vi "wavelength scan_v1.0.vi"() -> ()   [LabVIEW 2012]
panel:
  out "Power Chart":dbl(graph)=1.568e-05
  in  "range (0=auto)":i32
  in  "wavelength":i32=4
  in  "filter (0=out)":i32
  out "OfflineTEC_offset":dbl=-6.6023368 format="%#.4g"
  out "OnLineTEC_offset":dbl=-0.02357750000000003 format="%.4g"
  in  "offlineTEC_offset":dbl format="%.4g"
  in  "onlineTEC_offset":dbl format="%.4g"
  out "Lambda Read (nm)":dbl=780.2608522506264 format="%.5f"
  out "Wavelength Lock":bool=TRUE
  out "XY Graph":cluster{"Y":dbl[], "Y":dbl[]}[](graph)
  in  "Online":bool=TRUE
  out "Power (W)":dbl=1.568e-05 format="%.3p"
  out "OphirPM":T1={"Ophir-Ref"=refnum, "Ophir-Device"=1000, "Ophir-Channel"=0}
  out "Waveform Chart":dbl(graph)=780.2608522506264
  in  "Lambda Step (nm)":dbl=5e-05 format="%.5f"
  in  "Lambda Stop (nm)":dbl=780.261 format="%.5f"
  in  "Lambda Start (nm)":dbl=780.231 format="%.5f"
  in  "step_size":dbl=0.001 format="%#_6p"
  in  "Device In":refnum<visa-resource-name>="Pro8000"
  in  "Settings":T2={"Module"=enum."On Line TEC", "OnLineTEC"=14.05, "OnLineLD"=0.16, "OffLineTEC"=29.538, "OffLineLD"=0.173, "EtalonTEC"=27.0, "TSOA-TEC"=19.0} {"OffLineLD" min=0.0 max=0.175 step=0.001 format="%.3p"; "OnLineLD" min=0.0 max=0.175 step=0.001 format="%.3p"; "TSOA-TEC" format="%.2g"; "EtalonTEC" format="%.2g"; "OffLineTEC" min=0.0 max=30.0 step=0.1 format="%.3g"; "OnLineTEC" min=0.0 max=30.0 step=0.1 format="%.3g"}
  out "Readings":T3={"OnLineTEC"=14.0264225, "OnLineLD"=0.160541028, "OffLineTEC"=22.9356632, "OffLineLD"=0.000128906249, "EtalonTEC"=28.0260735, "TSOA-TEC"=19.0028629, "Pro8000"=TRUE, "OnLine TEC"=TRUE, "OnLine LD"=TRUE, "OffLine TEC"=FALSE, "OffLine LD"=FALSE, "Etalon TEC"=TRUE, "TSOA TEC"=TRUE} {"OffLineLD" format="%.4g"; "OnLineLD" format="%.4g"; "TSOA-TEC" format="%.3g"; "EtalonTEC" format="%.3g"; "OffLineTEC" format="%.3g"; "OnLineTEC" format="%.3g"}
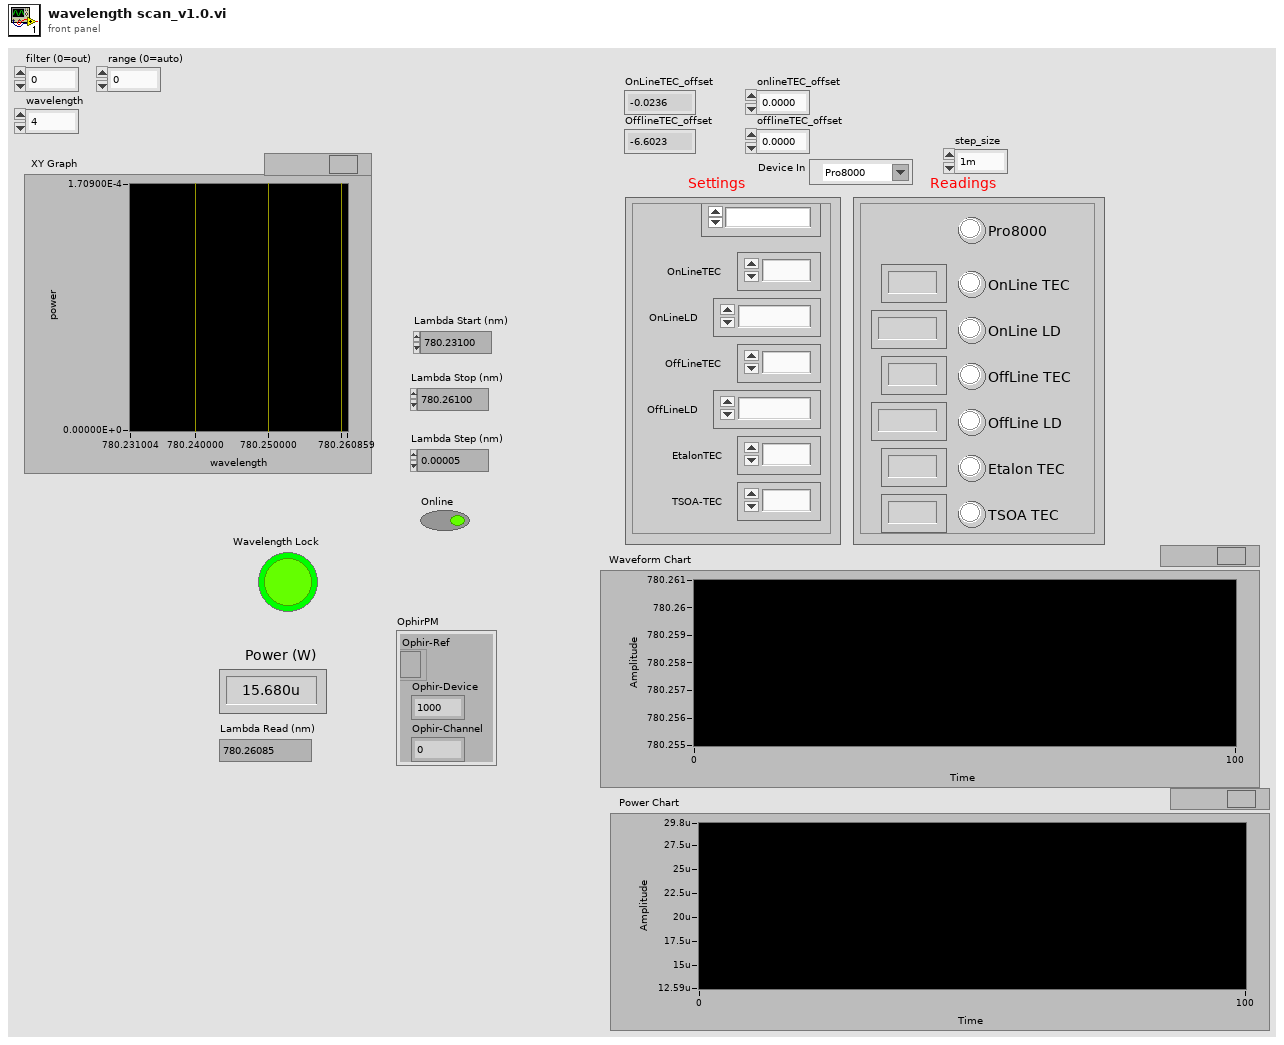
[diagram p1: front panel]
types:
  T1 = cluster{"Ophir-Ref":refnum<k7>, "Ophir-Device":i32, "Ophir-Channel":i32}
  T2 = cluster{"Module":enum16{"On Line TEC", "On Line LD", "Off Line TEC", "Off Line LD", "Etalon TEC", "TSOA TEC"}, "OnLineTEC":dbl, "OnLineLD":dbl, "OffLineTEC":dbl, "OffLineLD":dbl, "EtalonTEC":dbl, "TSOA-TEC":dbl}
  T3 = cluster{"OnLineTEC":dbl, "OnLineLD":dbl, "OffLineTEC":dbl, "OffLineLD":dbl, "EtalonTEC":dbl, "TSOA-TEC":dbl, "Pro8000":bool, "OnLine TEC":bool, "OnLine LD":bool, "OffLine TEC":bool, "OffLine LD":bool, "Etalon TEC":bool, "TSOA TEC":bool}
  T4 = enum16{"On Line TEC", "On Line LD", "Off Line TEC", "Off Line LD", "Etalon TEC", "TSOA TEC"}
  T5 = enum16{"Open_TL", "Close_TL", "Verify_ID", "TEC_Sensor", "SET", "READ", "ON", "OFF", "Set_Limits", "Read_Limits", "Enable_Status", "Read_Status"}
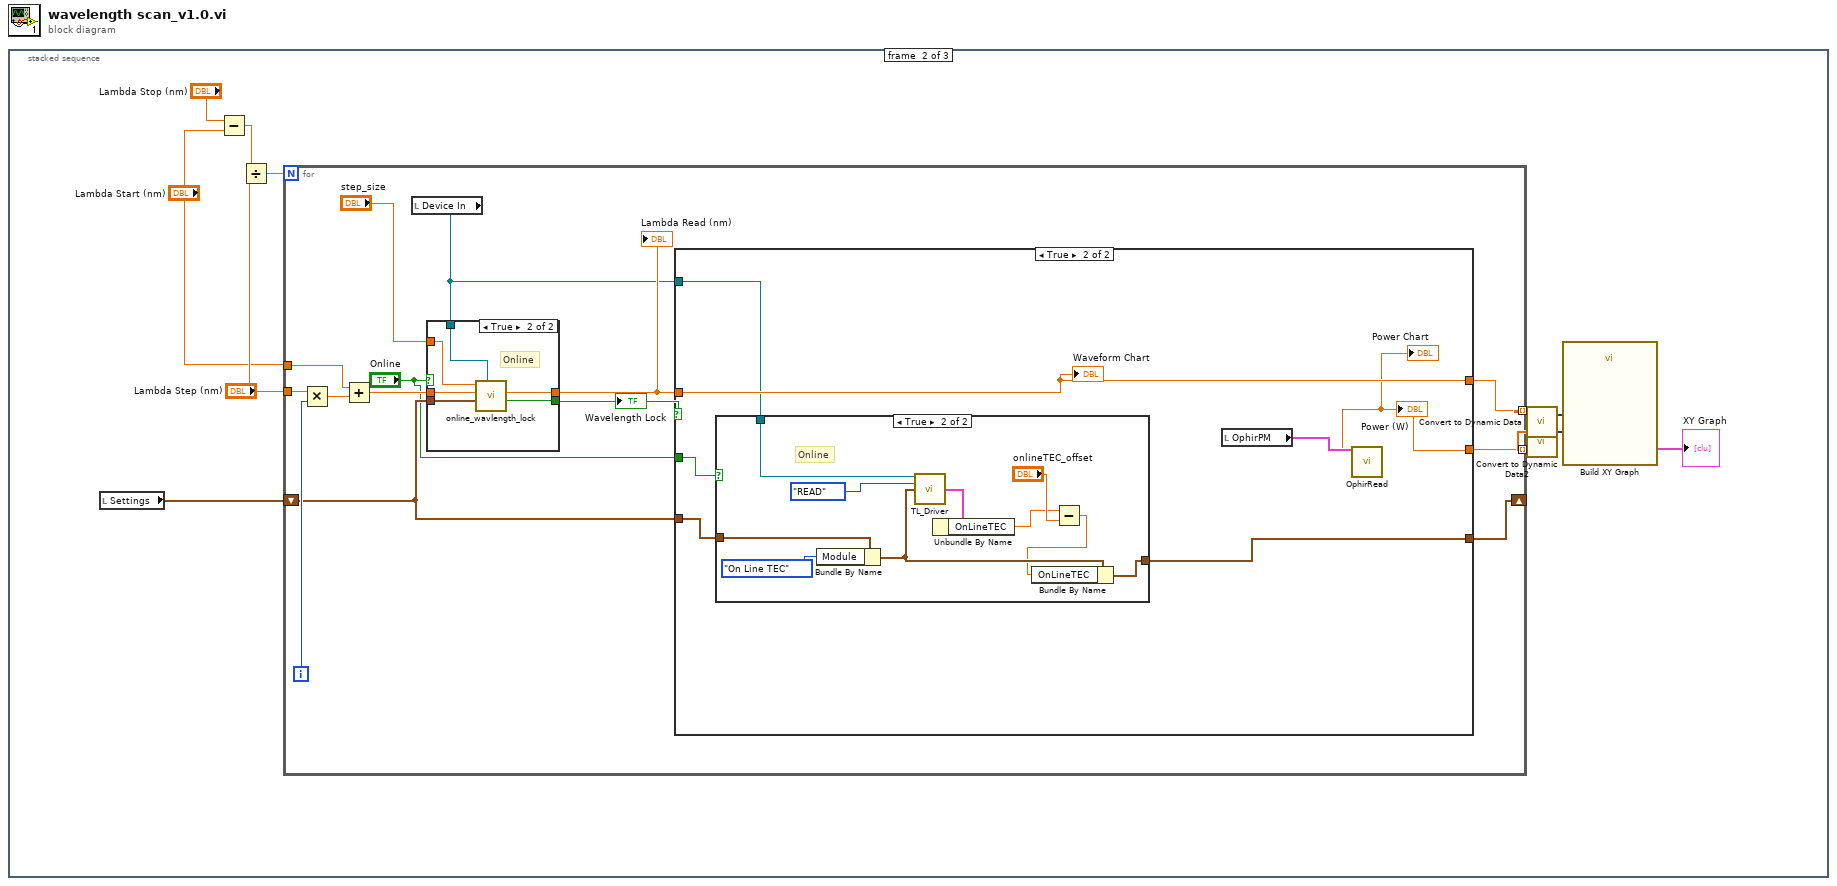
[diagram p0: block diagram]
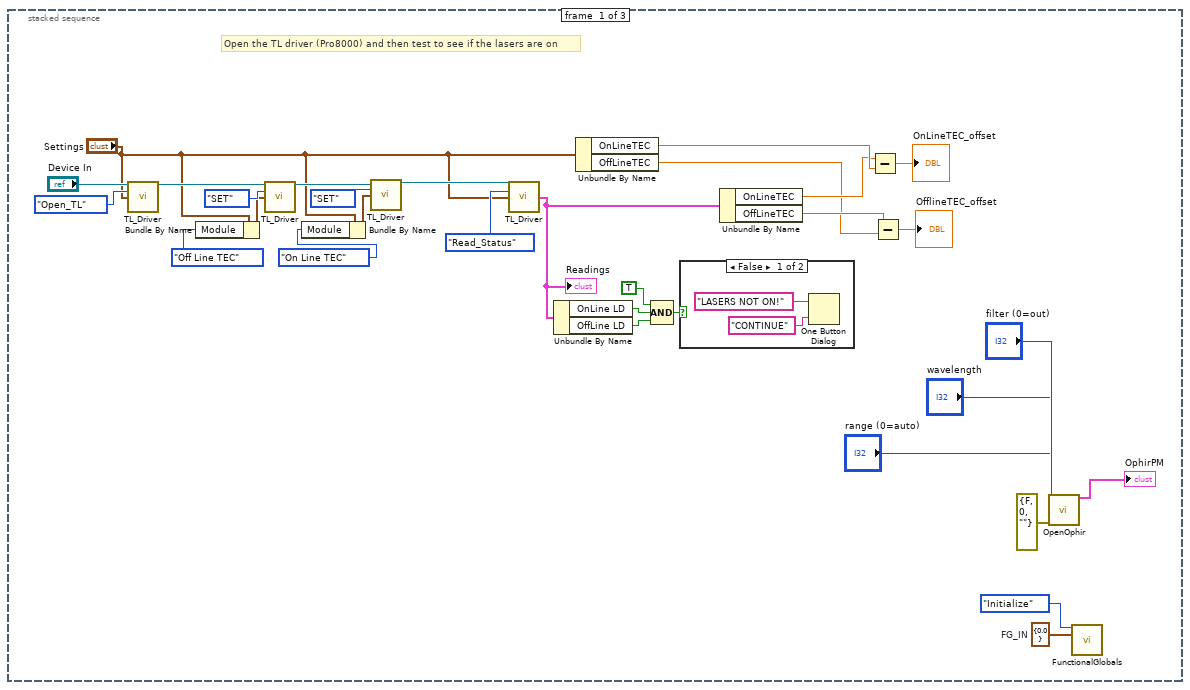
[diagram p2: hidden frame]
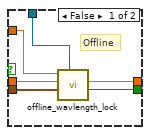
[diagram p4: hidden frame]
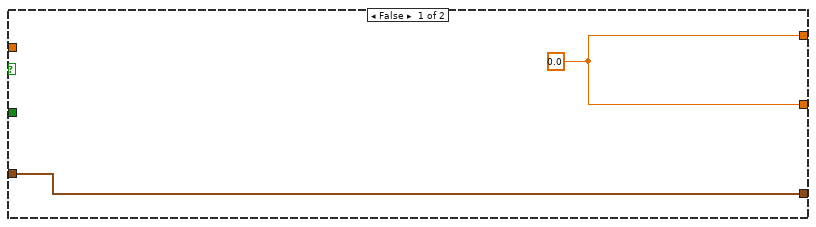
[diagram p5: hidden frame]
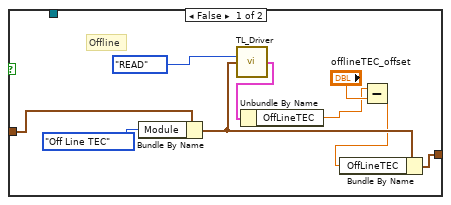
[diagram p6: hidden frame]
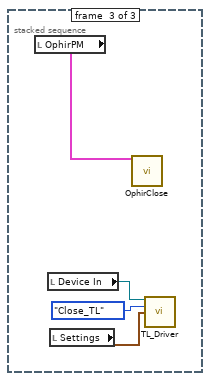
[diagram p7: hidden frame]
diagram:
  n1 = stacked-sequence {
    frame #0 {
      w22 = cluster{"PowerIn":dbl} {"PowerIn"=0.0}  # FG_IN
      # "Open the TL driver (Pro8000) and then test to see if the lasers are on"
      n2 = call "TL_Driver.vi"("Device In"="Device In", "Commands"=T5."Open_TL", "Settings"="Settings") -> ("Device Out"=w18:refnum<visa-resource-name>)  [unwired: 9 in, 3 out]
      n3 = Bundle By Name(cluster="Settings", "Module"=T4."Off Line TEC") -> (w15:T2)
      n4 = call "TL_Driver.vi"("Device In"=w18, "Commands"=T5."SET", "Settings"=w15) -> ("Device Out"=w13:refnum<visa-resource-name>)  [unwired: 9 in, 3 out]
      n5 = Bundle By Name(cluster="Settings", "Module"=T4."On Line TEC") -> (w14:T2)
      n6 = call "TL_Driver.vi"("Device In"=w13, "Commands"=T5."SET", "Settings"=w14) -> ("Device Out"=w12:refnum<visa-resource-name>)  [unwired: 9 in, 3 out]
      n7 = call "TL_Driver.vi"("Device In"=w12, "Commands"=T5."Read_Status", "Settings"="Settings") -> ("Readings"=w4:T3)  [unwired: 9 in, 3 out]
      "Readings" <- w4
      n8 = Unbundle By Name(w4) -> ("OnLine LD"=w29:bool, "OffLine LD"=w28:bool)
      n9 = Unbundle By Name("Settings") -> ("OnLineTEC"=w8:dbl, "OffLineTEC"=w5:dbl)
      n10 = Compound Arithmetic op=AND(TRUE, w29, w28) -> (w30:bool)
      n11 = case shown="False" w30 {
        frame False {
          n12 = One Button Dialog(message="LASERS NOT ON!", button name ("OK")="CONTINUE") -> ()  [unwired: 1 out]
        }
        frame True {
        }
      }
      n13 = Unbundle By Name(w4) -> ("OnLineTEC"=w7:dbl, "OffLineTEC"=w6:dbl)
      n14 = Subtract(x=w7, y=w8) -> (x-y=→"OnLineTEC_offset":dbl)
      n15 = Subtract(x=w6, y=w5) -> (x-y=→"OfflineTEC_offset":dbl)
      n16 = call "OpenOphir.vi"("filter (0=out)"="filter (0=out)", "wavelength"="wavelength", "range (0=auto)"="range (0=auto)", "error in (no error)"=errorcluster {"status"=FALSE, "code"=0, "source"=""}) -> ("OphirPM"=→"OphirPM":T1)  [unwired: 10 in, 1 out]
      n17 = call "FunctionalGlobals.vi"("FG_Control"=enum16{"Initialize", "PowerRead", "PowerWrite"}."Initialize", "FG_IN"=w22) -> ()  [unwired: 13 in, 1 out]
    }
    frame #1 {
      n18 = local read "Settings"() -> (w34:T2)
      n19 = Subtract(x="Lambda Stop (nm)", y="Lambda Start (nm)") -> (x-y=w44:dbl)
      n20 = Divide(x=w44, y="Lambda Step (nm)") -> (x/y=w43:dbl)
      n21 = for {
        N: w43 -> [_]
        tunnel: "Lambda Step (nm)" -> [w57]
        tunnel: "Lambda Start (nm)" -> [w56]
        tunnel: [w52] -> w38 mode=indexing
        tunnel: [w51] -> w36 mode=indexing
        shift-right: [w48] -> _
        shift-left: w34 -> [w46]
        i -> [w58]
        n22 = Multiply(x=w57, y=w58) -> (x*y=w55:dbl)
        n23 = Add(x=w56, y=w55) -> (x+y=w54:dbl)
        n24 = local read "Device In"() -> (w47:refnum<visa-resource-name>)
        n25 = case shown="True" "Online" {
          tunnel: w54 -> [w62 w70]
          tunnel: w47 -> [w63 w69]
          tunnel: w46 -> [w61 w68]
          tunnel: [w60 w67] -> w50
          tunnel: [w59 w66] -> w49
          tunnel: "step_size" -> [w64 w65]
          frame False {
            # "Offline"
            n26 = call "offline_wavlength_lock.vi"("Device"=w63, "Settings In"=w61, "Lambda Off Set (nm)"=w62, "step_size"=w64) -> ("Wavelength Lock Offline"=w60:bool, "Lambda Off Read (nm)"=w59:dbl)  [unwired: 3 in]
          }
          frame True {
            # "Online"
            n27 = call "online_wavlength_lock.vi"("Device"=w69, "Settings In"=w68, "Lambda On Set (nm)"=w70, "step_size"=w65) -> ("Wavelength Lock Online"=w67:bool, "Lambda On Read (nm)"=w66:dbl)  [unwired: 3 in]
          }
        }
        "Wavelength Lock" <- w50
        "Lambda Read (nm)" <- w49
        n28 = case shown="True" w50 {
          tunnel: w49 -> [_ w78]
          tunnel: [w72 w78] -> w52
          tunnel: [w72 w73] -> w51
          tunnel: [w71 w74] -> w48
          tunnel: w47 -> [_ w77]
          tunnel: w46 -> [w71 w76]
          tunnel: "Online" -> [_ w75]
          frame False {
            w72 = 0.0
          }
          frame True {
            n29 = case shown="True" w75 {
              tunnel: w77 -> [_ w97]
              tunnel: w76 -> [w87 w96]
              tunnel: [w83 w92] -> w74
              frame False {
                # "Offline"
                n30 = Bundle By Name(cluster=w87, "Module"=T4."Off Line TEC") -> (w84:T2)
                n31 = call "TL_Driver.vi"("Commands"=T5."READ", "Settings"=w84) -> ("Readings"=w85:T3)  [unwired: 10 in, 3 out]
                n32 = Unbundle By Name(w85) -> ("OffLineTEC"=w81:dbl)
                n33 = Subtract(x=w81, y="offlineTEC_offset") -> (x-y=w80:dbl)
                n34 = Bundle By Name(cluster=w84, "OffLineTEC"=w80) -> (w83:T2)
              }
              frame True {
                # "Online"
                n35 = Bundle By Name(cluster=w96, "Module"=T4."On Line TEC") -> (w93:T2)
                n36 = call "TL_Driver.vi"("Device In"=w97, "Commands"=T5."READ", "Settings"=w93) -> ("Readings"=w94:T3)  [unwired: 9 in, 3 out]
                n37 = Unbundle By Name(w94) -> ("OnLineTEC"=w90:dbl)
                n38 = Subtract(x=w90, y="onlineTEC_offset") -> (x-y=w89:dbl)
                n39 = Bundle By Name(cluster=w93, "OnLineTEC"=w89) -> (w92:T2)
              }
            }
            n40 = local read "OphirPM"() -> (w79:T1)
            n41 = call "OphirRead.vi"("OphirPM"=w79) -> ("Power (W)"=w73:dbl)  [unwired: 12 in, 2 out]
            "Power (W)" <- w73
            "Power Chart" <- w73
            "Waveform Chart" <- w78
          }
        }
      }
      n42 = call "Convert to Dynamic Data"("Array"=w38) -> ("Dynamic Data Type"=w37:dynamicdata)  [unwired: 3 in]
      n43 = call "Convert to Dynamic Data2"("Array"=w36) -> ("Dynamic Data Type"=w35:dynamicdata)  [unwired: 3 in]
      n44 = call "Build XY Graph"("Y Input"=w35, "X Input"=w37) -> ("XY Graph"=→"XY Graph":cluster{"Y":dbl[], "Y":dbl[]}[])  [unwired: 3 in, 6 out]
    }
    frame #2 {
      n45 = local read "OphirPM"() -> (w102:T1)
      n46 = local read "Device In"() -> (w99:refnum<visa-resource-name>)
      n47 = local read "Settings"() -> (w100:T2)
      n48 = call "OphirClose.vi"("OphirPM"=w102) -> ()  [unwired: 18 in, 1 out]
      n49 = call "TL_Driver.vi"("Device In"=w99, "Commands"=T5."Close_TL", "Settings"=w100) -> ()  [unwired: 9 in, 4 out]
    }
  }
